vi "Stop Modules.vi"(8 "error in (no error)":errorcluster, 9 "Message Queues in":T1) -> (0 "error out":errorcluster)   [LabVIEW 2020]
uses:
  Message Queue/All Message Queues.ctl
  Message Queue/Message Cluster.ctl
  MOTOR/Control Channel.ctl
  Message Queue/Enqueue Message (Single).vi
  Message Queue/Message Queue.lvlib
  MOTOR/MOTOR.lvlib
panel:
  in  "CMDs":string(combo)="ALARM"
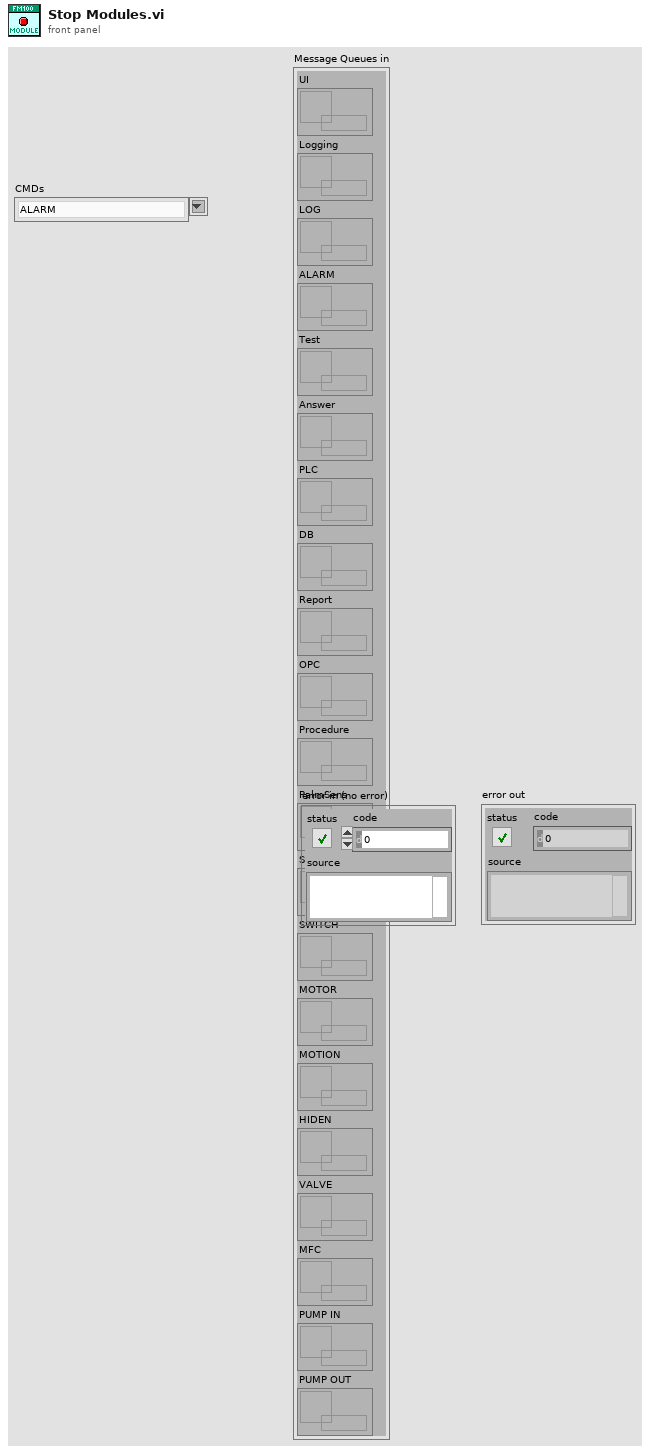
[diagram p1: front panel]
types:
  T1 = typedef "Message Queue.lvlib/All Message Queues.ctl" = cluster{"UI":refnum<queue>, "Logging":refnum<queue>, "LOG":refnum<queue>, "ALARM":refnum<queue>, "Test":refnum<queue>, "Answer":refnum<queue>, "PLC":refnum<queue>, "DB":refnum<queue>, "Report":refnum<queue>, "OPC":refnum<queue>, "Procedure":refnum<queue>, "PalmSens":refnum<queue>, "SYS 7000 Reader":refnum<queue>, "SWITCH":refnum<queue>, "MOTOR":refnum<queue>, "MOTION":refnum<queue>, "HIDEN":refnum<queue>, "VALVE":refnum<queue>, "MFC":refnum<queue>, "PUMP IN":refnum<queue>, "PUMP OUT":refnum<queue>}
  T2 = typedef "MOTOR.lvlib/Control Channel.ctl" = enum16{"Enable", "Manual Mode", "Jog Up", "Jog Down", "Set Zero Position", "Reset Error", "Move to Pos"}
  T3 = cluster{"Type CMD":string, "Mode CMD":string, "Main CMD":string}
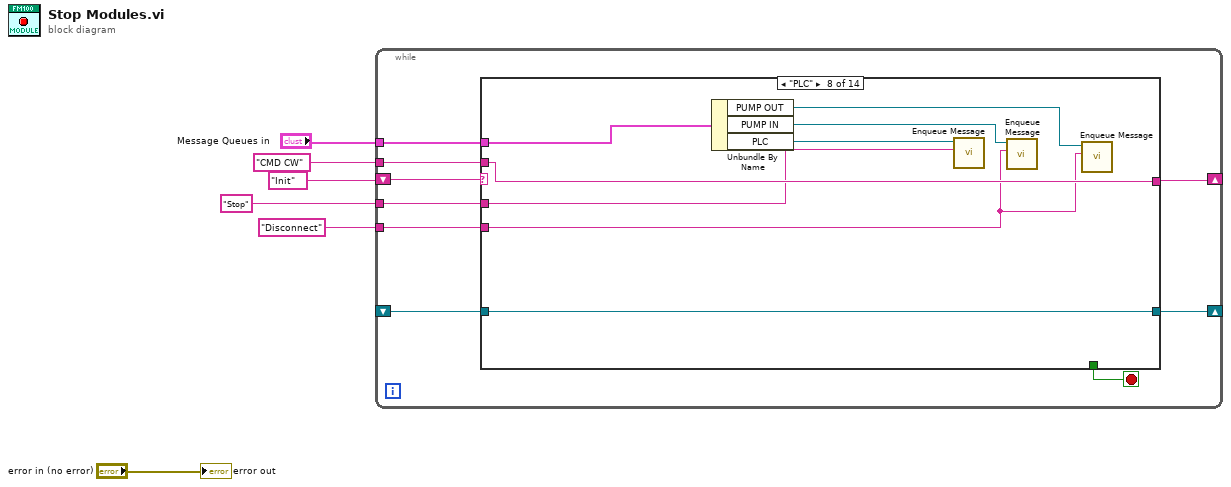
[diagram p0: block diagram]
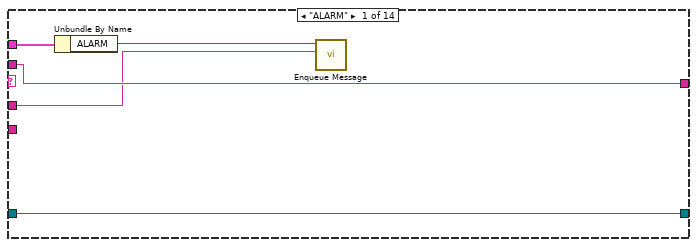
[diagram p2: hidden frame]
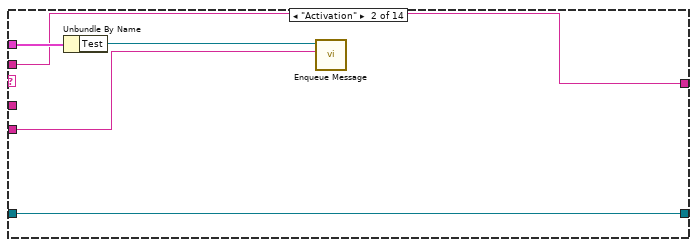
[diagram p3: hidden frame]
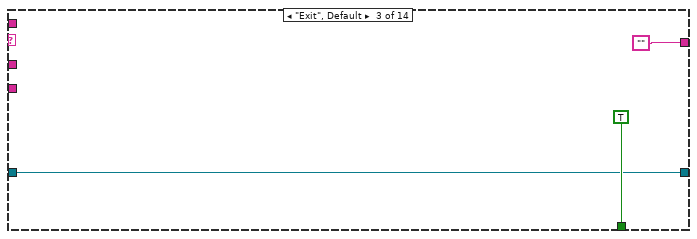
[diagram p4: hidden frame]
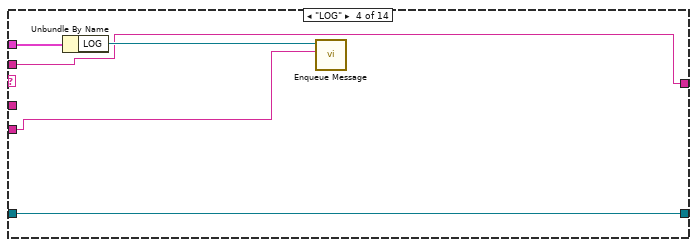
[diagram p5: hidden frame]
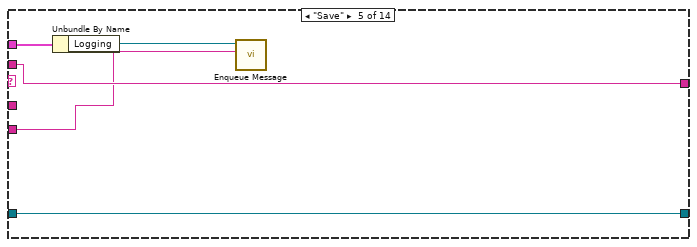
[diagram p6: hidden frame]
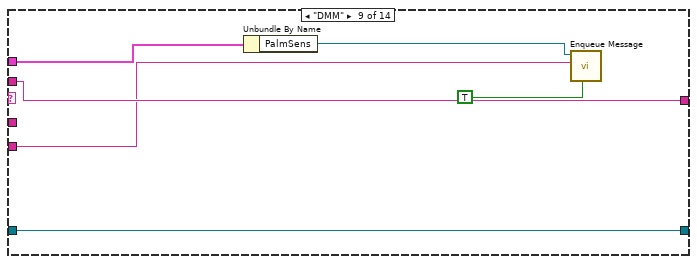
[diagram p9: hidden frame]
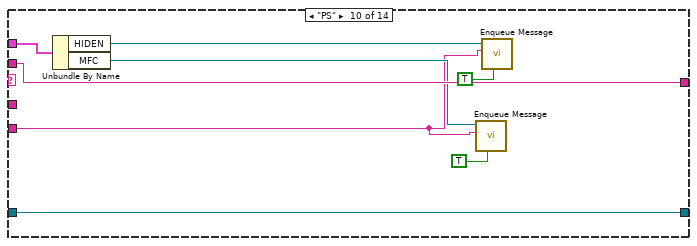
[diagram p10: hidden frame]
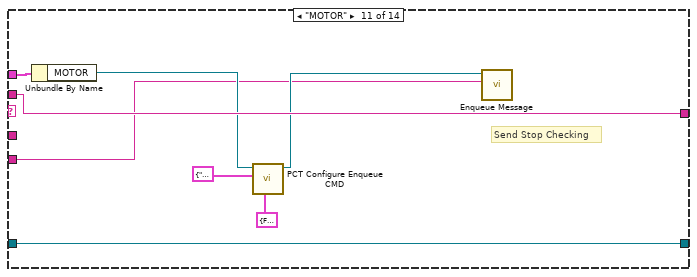
[diagram p11: hidden frame]
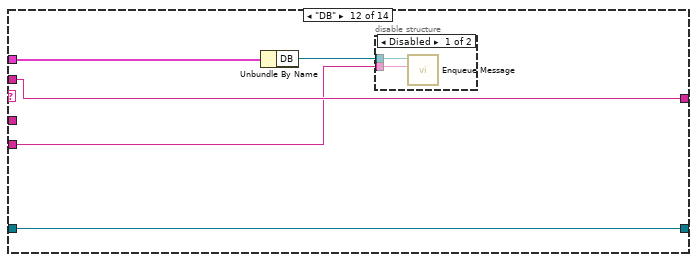
[diagram p12: hidden frame]
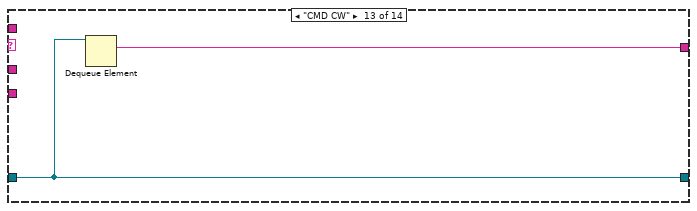
[diagram p14: hidden frame]
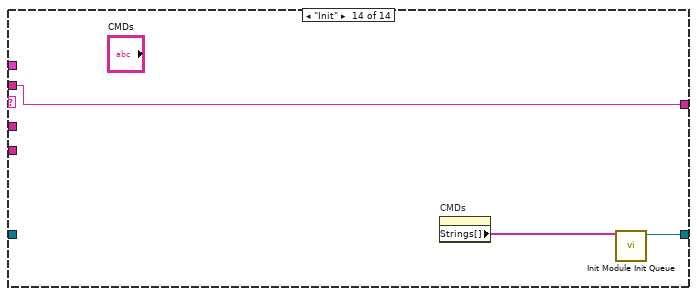
[diagram p15: hidden frame]
diagram:
  n1 = while {
    tunnel: "Message Queues in" -> [w14]
    tunnel: "Stop" ("Message") -> [w13]
    tunnel: "Disconnect" ("Message") -> [w12]
    shift-right: [w7] -> _
    shift-left: "Init" ("Combo Box") -> [w15]
    shift-right: [w9] -> _
    shift-left: _ -> [w10]
    tunnel: "CMD CW" ("Message") -> [w8]
    stop <- w11 stop-if-true
    n2 = case shown="\"PLC\"" w15 {
      tunnel: w14 -> [w20 w25 _ w33 w38 _ _ w50 w56 w64 w72 w77 _ _]
      tunnel: w13 -> [w16 _ _ _ _ _ _ w46 _ _ _ _ _ _]
      tunnel: w12 -> [_ w21 _ w32 w34 _ _ w43 w51 w57 w65 w73 _ _]
      tunnel: [w17 w22 "" w29 w35 w39 w41 w48 w54 w62 w70 w74 w80 w82] -> w7
      tunnel: [_ _ TRUE _ _ _ _ _ _ _ _ _ _ _] -> w11
      tunnel: [w18 w23 w26 w30 w36 w40 w42 w49 w55 w63 w71 w75 w81 w83] -> w9
      tunnel: w10 -> [w18 w23 w26 w30 w36 w40 w42 w49 w55 w63 w71 w75 w81 _]
      tunnel: w8 -> [w17 w22 _ w29 w35 w39 w41 w48 w54 w62 w70 w74 _ w82]
      frame "ALARM" {
        n3 = Unbundle By Name(w20) -> ("ALARM"=w19:refnum<queue>)
        n4 = call-poly "Enqueue Message.vi"("Message"=w16, "Message Queue"=w19) -> ()  [unwired: 8 in, 2 out]
      }
      frame "Activation" {
        n5 = Unbundle By Name(w25) -> ("Test"=w24:refnum<queue>)
        n6 = call-poly "Enqueue Message.vi"("Message"=w21, "Message Queue"=w24) -> ()  [unwired: 8 in, 2 out]
      }
      frame "Exit", Default {
      }
      frame "LOG" {
        n7 = Unbundle By Name(w33) -> ("LOG"=w31:refnum<queue>)
        n8 = call-poly "Enqueue Message.vi"("Message"=w32, "Message Queue"=w31) -> ()  [unwired: 8 in, 2 out]
      }
      frame "Save" {
        n9 = Unbundle By Name(w38) -> ("Logging"=w37:refnum<queue>)
        n10 = call-poly "Enqueue Message.vi"("Message"=w34, "Message Queue"=w37) -> ()  [unwired: 8 in, 2 out]
      }
      frame "PC Name" {
      }
      frame "SW Revision" {
      }
      frame "PLC" {
        n11 = Unbundle By Name(w50) -> ("PUMP OUT"=w44:refnum<queue>, "PUMP IN"=w45:refnum<queue>, "PLC"=w47:refnum<queue>)
        n12 = call-poly "Enqueue Message.vi"("Message"=w46, "Message Queue"=w47) -> ()  [unwired: 8 in, 2 out]
        n13 = call-poly "Enqueue Message.vi"("Message"=w43, "Message Queue"=w45) -> ()  [unwired: 8 in, 2 out]
        n14 = call-poly "Enqueue Message.vi"("Message"=w43, "Message Queue"=w44) -> ()  [unwired: 8 in, 2 out]
      }
      frame "DMM" {
        n15 = Unbundle By Name(w56) -> ("PalmSens"=w53:refnum<queue>)
        n16 = call-poly "Enqueue Message.vi"("Priority Message? (F)"=TRUE, "Message"=w51, "Message Queue"=w53) -> ()  [unwired: 7 in, 2 out]
      }
      frame "PS" {
        n17 = Unbundle By Name(w64) -> ("HIDEN"=w61:refnum<queue>, "MFC"=w58:refnum<queue>)
        n18 = call-poly "Enqueue Message.vi"("Priority Message? (F)"=TRUE, "Message"=w57, "Message Queue"=w58) -> ()  [unwired: 7 in, 2 out]
        n19 = call-poly "Enqueue Message.vi"("Priority Message? (F)"=TRUE, "Message"=w57, "Message Queue"=w61) -> ()  [unwired: 7 in, 2 out]
      }
      frame "MOTOR" {
        # "Send Stop Checking"
        n20 = Unbundle By Name(w72) -> ("MOTOR"=w67:refnum<queue>)
        n21 = call "PCT Configure Enqueue CMD.vi"("Parameter Data"=cluster{"Status":bool, "Channel":T2} {"Status"=FALSE, "Channel"=enum."Enable"}, "CMD"=T3 {"Type CMD"="Control", "Mode CMD"="", "Main CMD"="Configure"}, "CMD Queue in"=w67) -> ("CMD Queue out"=w66:refnum<queue>)  [unwired: 6 in, 2 out]
        n22 = call-poly "Enqueue Message.vi"("Message"=w65, "Message Queue"=w66) -> ()  [unwired: 8 in, 2 out]
      }
      frame "DB" {
        n23 = Unbundle By Name(w77) -> ("DB"=w76:refnum<queue>)
        n24 = disable-structure shown="Disabled" {
          disable-tunnel: w76 -> [w79 _]
          disable-tunnel: w73 -> [w78 _]
          frame Disabled {
            n25 = call-poly "Enqueue Message.vi"("Message"=w78, "Message Queue"=w79) -> ()  [unwired: 8 in, 2 out]
          }
          frame Enabled {
          }
        }
      }
      frame "CMD CW" {
        n26 = Dequeue Element(queue=w81) -> (element=w80:string)  [unwired: 2 in, 3 out]
      }
      frame "Init" {
        n27 = property on="CMDs" class="CmbBox"() -> ("Strings[]"=w84:string[])  [unwired: 2 in, 2 out]
        n28 = call "Init Module Init Queue.vi"("Strings[]"=w84) -> ("Queue out"=w83:refnum<queue>)  [unwired: 10 in]
      }
    }
  }
  "error out" <- "error in (no error)"
